vi "Measure Element.vi"(8 "error in (no error)":errorcluster, 10 "Element (1: Element 1)":u16(ring)=1 items=["", "Element1", "Element2", "Element3", "Sigma"], 11 "VISA resource name":refnum<visa-resource-name>) -> (0 "error out":errorcluster, 2 "Array":string[][](array[string]), 3 "VISA resource name out":refnum<visa-resource-name>)   [LabVIEW 2014, in "Generic Power Analyzer.lvlib" / "Yokogawa WT2X0.lvlib" / "Yokogawa WT2X0.lvclass"]
uses:
  Yokogawa WT2X0.lvclass
  <instrlib>/Yokogawa WT200 Series/Yokogawa WT200 Series.lvlib
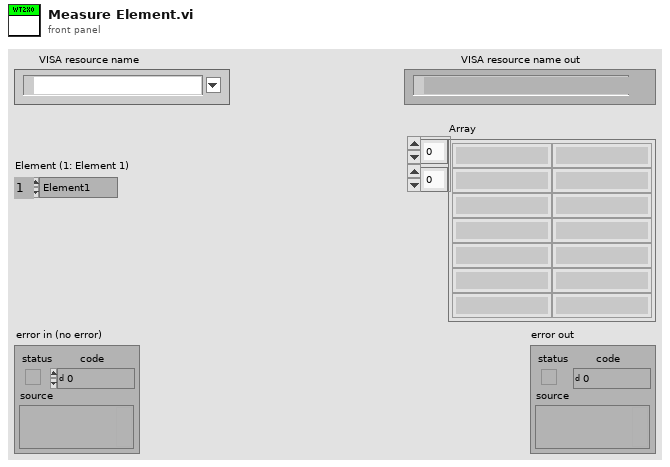
[diagram p1: front panel]
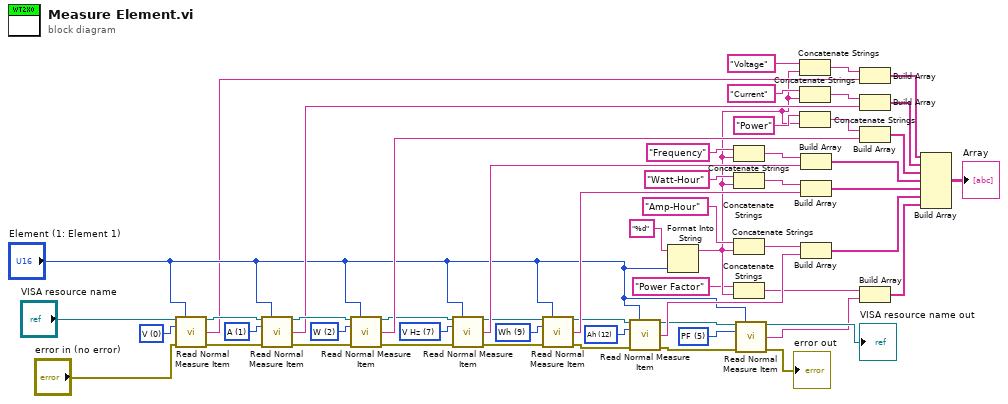
[diagram p0: block diagram]
diagram:
  w7 = u16 5 items=["V", "A", "W", "VA", "var", "PF", "deg", "V Hz", "A Hz", "Wh", "Wh+", "Wh-", "Ah", "Ah+", "Ah-", "Vpk", "Apk", "Math"] ("Measure Item (0: V)")
  w14 = u16 12 items=["V", "A", "W", "VA", "var", "PF", "deg", "V Hz", "A Hz", "Wh", "Wh+", "Wh-", "Ah", "Ah+", "Ah-", "Vpk", "Apk", "Math"] ("Measure Item (0: V)")
  w24 = u16 9 items=["V", "A", "W", "VA", "var", "PF", "deg", "V Hz", "A Hz", "Wh", "Wh+", "Wh-", "Ah", "Ah+", "Ah-", "Vpk", "Apk", "Math"] ("Measure Item (0: V)")
  w32 = u16 7 items=["V", "A", "W", "VA", "var", "PF", "deg", "V Hz", "A Hz", "Wh", "Wh+", "Wh-", "Ah", "Ah+", "Ah-", "Vpk", "Apk", "Math"] ("Measure Item (0: V)")
  w44 = u16 2 items=["V", "A", "W", "VA", "var", "PF", "deg", "V Hz", "A Hz", "Wh", "Wh+", "Wh-", "Ah", "Ah+", "Ah-", "Vpk", "Apk", "Math"] ("Measure Item (0: V)")
  w47 = u16 1 items=["V", "A", "W", "VA", "var", "PF", "deg", "V Hz", "A Hz", "Wh", "Wh+", "Wh-", "Ah", "Ah+", "Ah-", "Vpk", "Apk", "Math"] ("Measure Item (0: V)")
  w54 = u16 0 items=["V", "A", "W", "VA", "var", "PF", "deg", "V Hz", "A Hz", "Wh", "Wh+", "Wh-", "Ah", "Ah+", "Ah-", "Vpk", "Apk", "Math"] ("Measure Item (0: V)")
  n1 = call <instrlib>:"Read Normal Measure Item.vi"("VISA resource name"="VISA resource name", "Element (1: Element 1)"="Element (1: Element 1)", "Measure Item (0: V)"=w54, "error in (no error)"="error in (no error)") -> ("VISA resource name out"=w53:refnum<visa-resource-name>, "Measured Value"=w5:string, "error out"=w49:errorcluster)  [unwired: 8 in, 1 out]
  n2 = call <instrlib>:"Read Normal Measure Item.vi"("VISA resource name"=w53, "Element (1: Element 1)"="Element (1: Element 1)", "Measure Item (0: V)"=w47, "error in (no error)"=w49) -> ("VISA resource name out"=w46:refnum<visa-resource-name>, "Measured Value"=w41:string, "error out"=w45:errorcluster)  [unwired: 8 in, 1 out]
  n3 = call <instrlib>:"Read Normal Measure Item.vi"("VISA resource name"=w46, "Element (1: Element 1)"="Element (1: Element 1)", "Measure Item (0: V)"=w44, "error in (no error)"=w45) -> ("VISA resource name out"=w33:refnum<visa-resource-name>, "Measured Value"=w37:string, "error out"=w31:errorcluster)  [unwired: 8 in, 1 out]
  n4 = call <instrlib>:"Read Normal Measure Item.vi"("VISA resource name"=w33, "Element (1: Element 1)"="Element (1: Element 1)", "Measure Item (0: V)"=w32, "error in (no error)"=w31) -> ("VISA resource name out"=w26:refnum<visa-resource-name>, "Measured Value"=w29:string, "error out"=w25:errorcluster)  [unwired: 8 in, 1 out]
  n5 = call <instrlib>:"Read Normal Measure Item.vi"("VISA resource name"=w26, "Element (1: Element 1)"="Element (1: Element 1)", "Measure Item (0: V)"=w24, "error in (no error)"=w25) -> ("VISA resource name out"=w19:refnum<visa-resource-name>, "Measured Value"=w21:string, "error out"=w18:errorcluster)  [unwired: 8 in, 1 out]
  n6 = call <instrlib>:"Read Normal Measure Item.vi"("VISA resource name"=w19, "Element (1: Element 1)"="Element (1: Element 1)", "Measure Item (0: V)"=w14, "error in (no error)"=w18) -> ("VISA resource name out"=w11:refnum<visa-resource-name>, "Measured Value"=w15:string, "error out"=w9:errorcluster)  [unwired: 8 in, 1 out]
  n7 = Format Into String(format string="%d", "Element (1: Element 1)") -> (resulting string=w3:string)  [unwired: 2 in, 1 out]
  n8 = Concatenate Strings("Frequency" ("string"), w3) -> (w28:string)
  n9 = Concatenate Strings("Watt-Hour" ("string"), w3) -> (w23:string)
  n10 = Concatenate Strings("Amp-Hour" ("string"), w3) -> (w16:string)
  n11 = Concatenate Strings("Power Factor" ("string"), w3) -> (w6:string)
  n12 = call <instrlib>:"Read Normal Measure Item.vi"("VISA resource name"=w11, "Element (1: Element 1)"="Element (1: Element 1)", "Measure Item (0: V)"=w7, "error in (no error)"=w9) -> ("VISA resource name out"=→"VISA resource name out":refnum<visa-resource-name>, "Measured Value"=w4:string, "error out"=→"error out":errorcluster)  [unwired: 8 in, 1 out]
  n13 = Concatenate Strings("Voltage" ("string"), w3) -> (w51:string)
  n14 = Concatenate Strings("Current" ("string"), w3) -> (w43:string)
  n15 = Concatenate Strings("Power" ("string"), w3) -> (w35:string)
  n16 = Build Array(w28, w29) -> (w27:string[])
  n17 = Build Array(w23, w21) -> (w20:string[])
  n18 = Build Array(w16, w15) -> (w13:string[])
  n19 = Build Array(w51, w5) -> (w42:string[])
  n20 = Build Array(w43, w41) -> (w39:string[])
  n21 = Build Array(w35, w37) -> (w34:string[])
  n22 = Build Array(w6, w4) -> (w1:string[])
  n23 = Build Array(w42, w39, w34, w27, w20, w13, w1) -> (→"Array":string[][])
